vi "write_data_kn.vi"(8 "error in (no error)":errorcluster, 10 "data+":T1={"n_neighbors"=0.0, "mode"="connectivity", "return_distance"=TRUE}, 11 "KNeighbors in":refnum<class "KNeighbors.lvclass">) -> (0 "error out":errorcluster, 3 "KNeighbors out":refnum<class "KNeighbors.lvclass">)   [LabVIEW 2020, in "KNeighbors.lvclass"]
uses:
  KNeighbors.lvclass
  Controls/kneighbors_data.ctl
  KNeighbors.lvclass/KNeighbors.ctl
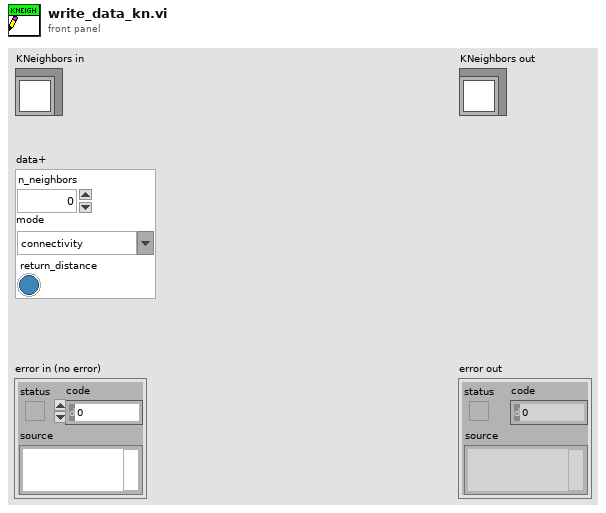
[diagram p1: front panel]
types:
  T1 = typedef "kneighbors_data.ctl" = cluster{"n_neighbors":dbl, "mode":string, "return_distance":bool}
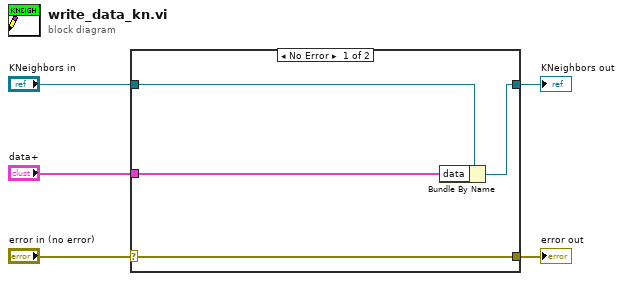
[diagram p0: block diagram]
diagram:
  n1 = case shown="No Error" "error in (no error)" {
    selector: "error in (no error)" -> [w9 w10]
    tunnel: [w9 w10] -> w4
    tunnel: [w7 w11] -> w2
    tunnel: "KNeighbors in" -> [w8 w11]
    tunnel: "data+" -> [w6 _]
    frame No Error {
      n2 = Bundle By Name(cluster=w8, "data"=w6) -> (w7:refnum<class "KNeighbors.lvclass">)
    }
    frame Error {
    }
  }
  "error out" <- w4
  "KNeighbors out" <- w2
